vi "Autosetup.vi"(6 "Auto Scale Acquisition Type (0: Normal)":i32(ring) items=["Normal", "Current"], 7 "Auto Scale Source (0: Channel 1)":i32(ring) items=["Channel 1"=0, "Channel 2"=1, "Channel 3"=2, "Channel 4"=3, "Digital Bus Low"=9, "Digital Bus High"=10], 8 "error in (no error)":errorcluster, 9 "Enable Fast Debug Auto Scaling (F: Disable)":bool, 10 "Auto Scale Channel (0: All)":i32(ring) items=["All", "Displayed"], 11 "VISA resource name":refnum<visa-resource-name>) -> (0 "error out":errorcluster, 3 "VISA resource name out":refnum<visa-resource-name>)   [LabVIEW 2015, in "Agilent 2000 3000 X-Series.lvlib"]
doc: "Causes the oscilloscope to evaluate all input waveforms and find the optimum conditions for displaying the waveform.\n\n<B>Note(s):</B> \nAutosetup sets the instrument in continuous acquisition mode."
uses:
  <instrlib>/Agilent 2000 3000 X-Series/Agilent 2000 3000 X-Series.lvlib
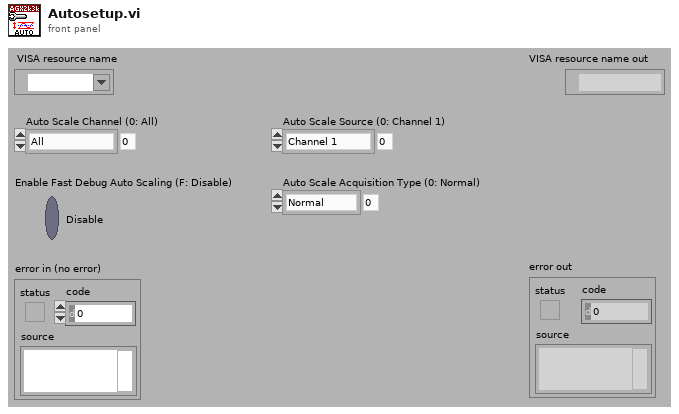
[diagram p1: front panel]
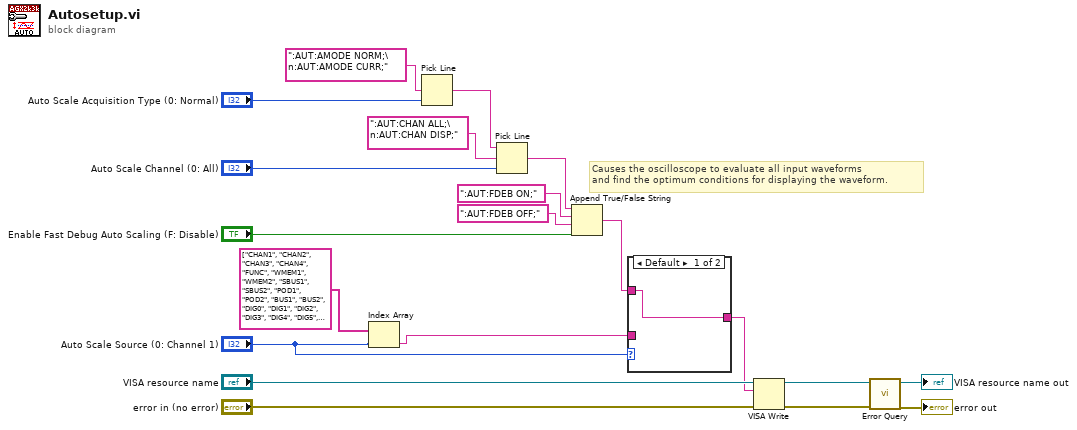
[diagram p0: block diagram]
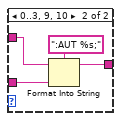
[diagram p2: hidden frame]
diagram:
  # "Causes the oscilloscope to evaluate all input waveforms \nand find the optimum conditions for displaying the waveform."
  n1 = Index Array(array=string[] ["CHAN1", "CHAN2", "CHAN3", "CHAN4", "FUNC", "WMEM1", "WMEM2", "SBUS1", "SBUS2", "POD1", "POD2", "BUS1", "BUS2", "DIG0", "DIG1", "DIG2", "DIG3", "DIG4", "DIG5", "DIG6", "DIG7", "DIG8", "DIG9", "DIG10", "DIG11", "DIG12", "DIG13", "DIG14", "DIG15", "EXT", "LINE", "WGEN"], index="Auto Scale Source (0: Channel 1)") -> (element=w3:string)
  n2 = Pick Line(multi-line string=":AUT:AMODE NORM;\n:AUT:AMODE CURR;", line index="Auto Scale Acquisition Type (0: Normal)") -> (output string=w16:string)  [unwired: 1 out]
  n3 = Pick Line(string ("")=w16, multi-line string=":AUT:CHAN ALL;\n:AUT:CHAN DISP;", line index="Auto Scale Channel (0: All)") -> (output string=w15:string)
  n4 = Append True/False String(1:"Enable Fast Debug Auto Scaling (F: Disable)", 2:":AUT:FDEB OFF;", 3:":AUT:FDEB ON;", 4:w15) -> (0:w5:string)
  n5 = case shown="Default" "Auto Scale Source (0: Channel 1)" {
    tunnel: w5 -> [w21 w24]
    tunnel: [w21 w23] -> w4
    tunnel: w3 -> [_ w22]
    frame Default {
    }
    frame 0..3, 9, 10 {
      n6 = Format Into String(format string=":AUT %s;", initial string=w24, w22) -> (resulting string=w23:string)  [unwired: 1 in, 1 out]
    }
  }
  n7 = VISA Write(VISA resource name="VISA resource name", write buffer=w4, error in (no error)="error in (no error)") -> (VISA resource name out=w9:refnum<visa-resource-name>, error out=w8:errorcluster)  [unwired: 1 out]
  n8 = call <instrlib>:"Error Query.vi"("error in (no error)"=w8, "VISA resource name"=w9) -> ("error out"=→"error out":errorcluster, "VISA resource name out"=→"VISA resource name out":refnum<visa-resource-name>)  [unwired: 8 out]
